vi "main.vi"() -> ()   [LabVIEW 2016]
uses:
  <userlib>/ROS for LabVIEW Software/ROS/Code/Console/Servers/ServerSubs/TopicDef.ctl
  <userlib>/ROS for LabVIEW Software/ROS/Code/SubVIs/_ROSDirection.ctl
  <userlib>/ROS for LabVIEW Software/ROS/MessageBuilding/std_msgs/subs/i8Scalar.vi
panel:
  in  "EM STOP":bool
  out "error out":errorcluster
  out "time":T1
  out "Error":cluster{"Error Code":i8, "Error Message":string}
  out "Ultrasonics":T2
  out "Lasers":T2
  in  "stop":bool
  out "Velocity":dbl
  out "Steering Angle":dbl(knob) scale=-20.0..20.0
  in  "settings":T3={"Enable"=0, "Run"=0, "GUI Connection"=1, "Max Speed"=3.0} {"Max Speed" min=0.5 max=10.0 step=0.25}
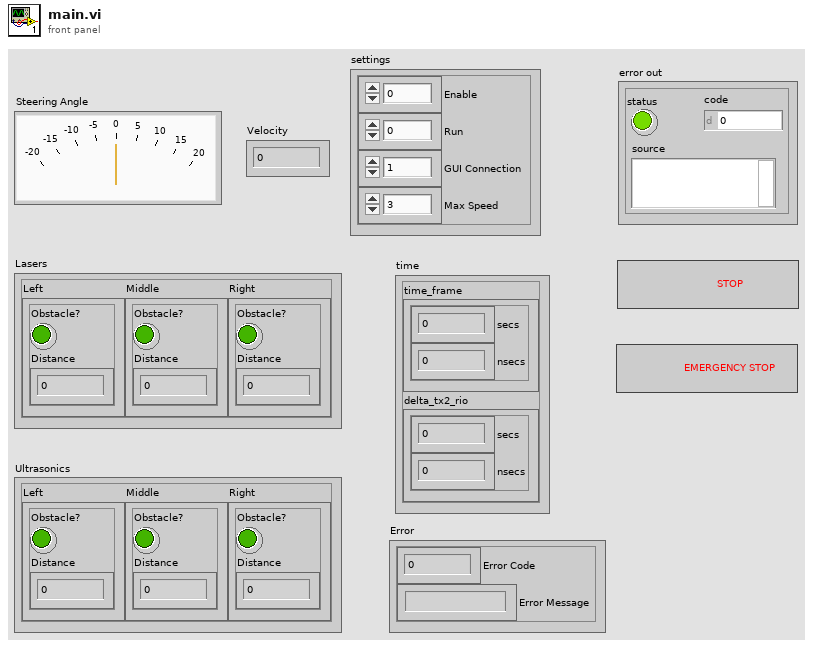
[diagram p1: front panel]
types:
  T1 = cluster{"time_frame":cluster{"secs":dbl, "nsecs":dbl}, "delta_tx2_rio":cluster{"secs":dbl, "nsecs":dbl}}
  T2 = cluster{"Left":cluster{"Obstacle?":bool, "Distance":dbl}, "Middle":cluster{"Obstacle?":bool, "Distance":dbl}, "Right":cluster{"Obstacle?":bool, "Distance":dbl}}
  T3 = cluster{"Enable":i8, "Run":i8, "GUI Connection":i8, "Max Speed":dbl}
  T4 = typedef "TopicDef.ctl" = cluster{"Topic":string, "Type":string, "Action":T5, "Update (ms)":u16, "queue size":u16}
  T5 = typedef "_ROSDirection.ctl" = enum16{"Node", "Publisher", "Subscriber", "ServiceClient", "ServiceProvider"}
  T6 = typedef "_ROSControl.ctl" = cluster{"topic port":u16, "Node":string, "topic":string, "type":string, "node port":u16, "error ":errorcluster, "Direction":T5, "Update (ms)":u16, "FIFO size":u16}
  T7 = cluster{"time_frame":cluster{"secs":i32, "nsecs":i32}, "delta_tx2_rio":cluster{"secs":i32, "nsecs":i32}}
  T8 = cluster{"speed_is":cluster{"steering_front_left":dbl, "steering_front_right":dbl, "steering_rear_left":dbl, "steering_rear_right":dbl}, "steering_is":cluster{"steering_front_left":dbl, "steering_front_right":dbl, "steering_rear_left":dbl, "steering_rear_right":dbl}, "distance_front":cluster{"left":dbl, "middle":dbl, "right":dbl}, "distance_back":cluster{"left":dbl, "middle":dbl, "right":dbl}, "error_id":i8, "error_message":string, "time_frame":cluster{"secs":i32, "nsecs":i32}, "delta_tx2_rio":cluster{"secs":i32, "nsecs":i32}}
  T9 = cluster{"steering_front_left":dbl, "steering_front_right":dbl, "steering_rear_left":dbl, "steering_rear_right":dbl}
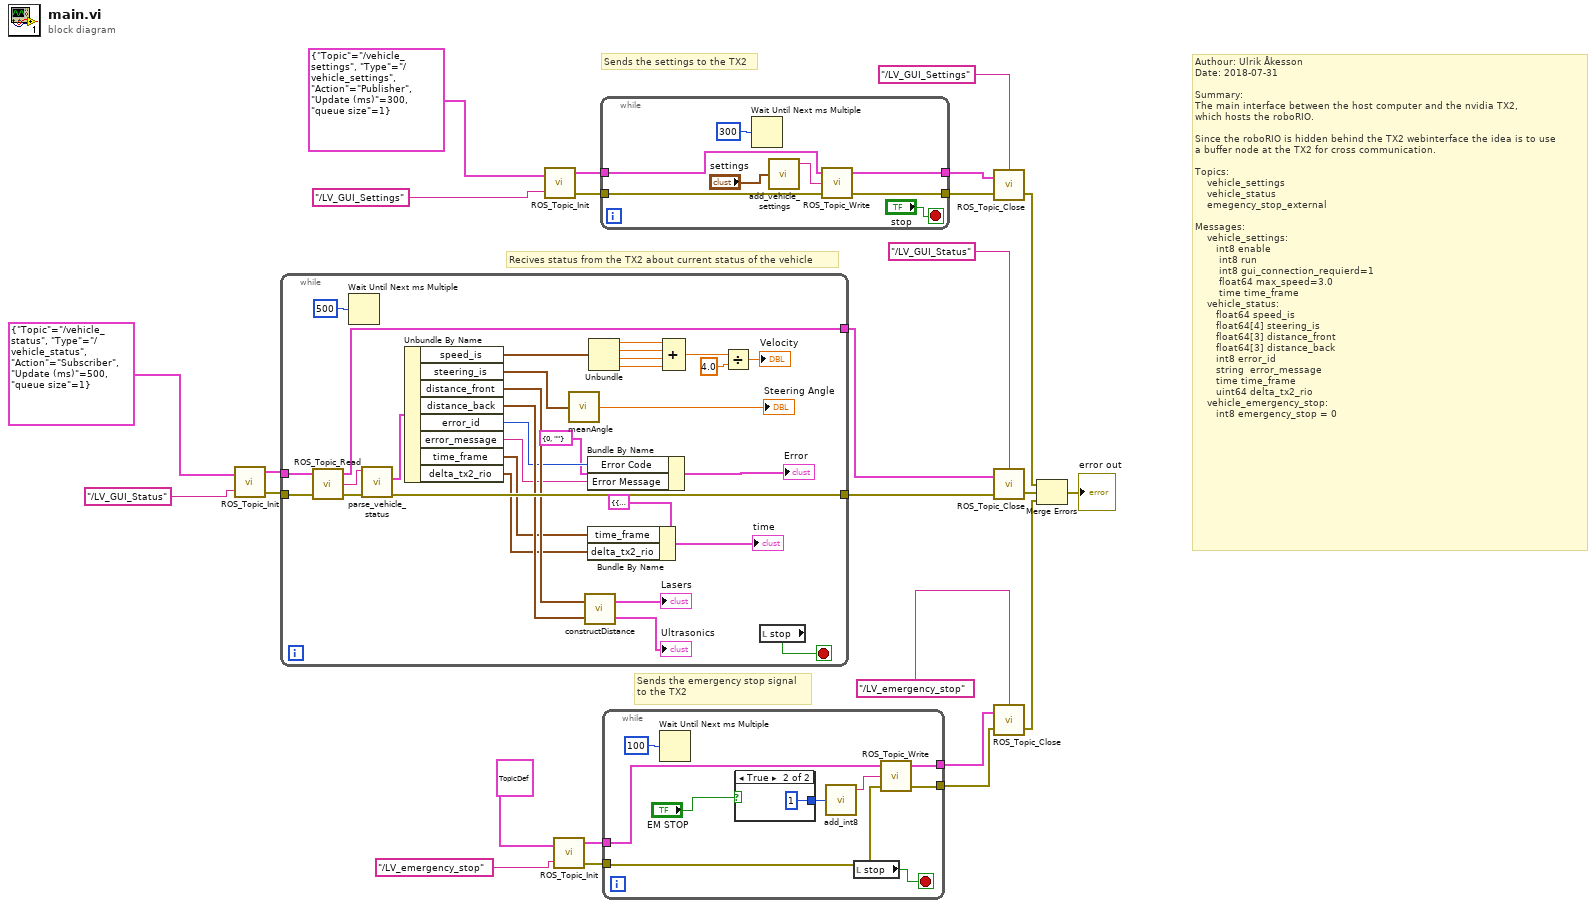
[diagram p0: block diagram]
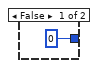
[diagram p2: hidden frame]
diagram:
  # "Sends the emergency stop signal\nto the TX2"
  # "Recives status from the TX2 about current status of the vehicle"
  # "Sends the settings to the TX2"
  # "Authour: Ulrik Åkesson\nDate: 2018-07-31\n\nSummary:\nThe main interface between the host computer and the nvidia TX2,\nwhich hosts the roboRIO.\n\nSince the roboRIO is hidden behind the TX2 webinterface the idea is to use\na buffer node at the TX2 for cross communication.\n\nTopics:\n    vehicle_settings\n    vehicle_status\n    emegency_stop_external\n\nMessages:\n    vehicle_settings:\n       int8 enable\n        int8 run\n        int8 gui_connection_requierd=1\n        float64 max_speed=3.0\n        time time_frame \n    vehicle_status:\n       float64 speed_is\n       float64[4] steering_is\n       float64[3] distance_front\n       float64[3] distance_back\n       int8 error_id\n       string  error_message\n       time time_frame\n       uint64 delta_tx2_rio\n    vehicle_emergency_stop:\n       int8 emergency_stop = 0"
  n1 = call <userlib>:"ROS_Topic_Init.vi"("Definitions"=T4 {"Topic"="/vehicle_status", "Type"="/vehicle_status", "Action"=enum."Subscriber", "Update (ms)"=500, "queue size"=1}, "node"="/LV_GUI_Status") -> ("ROS out"=w16:T6, "error out"=w15:errorcluster)  [unwired: 1 in]
  n2 = while {
    tunnel: w16 -> [w56]
    tunnel: w15 -> [w55]
    tunnel: [w50] -> w13
    tunnel: [w51] -> w12
    stop <- w49 stop-if-true
    n3 = call <userlib>:"ROS_Topic_Read.vi"("error in (no error)"=w55, "ROS in"=w56) -> ("error out"=w53:errorcluster, "Reply"=w54:string, "ROS out"=w50:T6)  [unwired: 1 in]
    n4 = Wait Until Next ms Multiple(millisecond multiple=u32 500) -> ()  [unwired: 1 out]
    n5 = call "parse_vehicle_status.vi"("error in"=w53, "msg in"=w54) -> ("error out"=w51:errorcluster, "vehicle_status"=w52:T8)  [unwired: 7 in, 1 out]
    n6 = Unbundle By Name(w52) -> ("speed_is"=w33:T9, "steering_is"=w47:T9, "distance_front"=w46:cluster{"left":dbl, "middle":dbl, "right":dbl}, "distance_back"=w45:cluster{"left":dbl, "middle":dbl, "right":dbl}, "error_id"=w42:i8, "error_message"=w41:string, "time_frame"=w37:cluster{"secs":i32, "nsecs":i32}, "delta_tx2_rio"=w36:cluster{"secs":i32, "nsecs":i32})
    n7 = call "meanAngle.vi"("steering_is"=w47) -> ("Numeric"=→"Steering Angle":dbl)
    n8 = call "constructDistance.vi"("distance_front"=w45, "distance_back"=w46) -> ("Ultrasonics"=→"Ultrasonics":T2, "Lasers"=→"Lasers":T2)
    n9 = Bundle By Name(cluster=cluster{"Error Code":i8, "Error Message":string} {"Error Code"=0, "Error Message"=""} ("Error 2"), "Error Code"=w42, "Error Message"=w41) -> (→"Error":cluster{"Error Code":i8, "Error Message":string})
    n10 = Bundle By Name(cluster=T7 {"time_frame"={"secs"=0, "nsecs"=0}, "delta_tx2_rio"={"secs"=0, "nsecs"=0}}, "time_frame"=w37, "delta_tx2_rio"=w36) -> (→"time":T7)
    n11 = Unbundle(w33) -> ("steering_front_left"=w32:dbl, "steering_front_right"=w31:dbl, "steering_rear_left"=w30:dbl, "steering_rear_right"=w29:dbl)
    n12 = Compound Arithmetic op=ADD(w32, w31, w30, w29) -> (w27:dbl)
    n13 = Divide(x=w27, y=4.0) -> (x/y=→"Velocity":dbl)
    n14 = local read "stop"() -> (w49:bool)
  }
  n15 = call <userlib>:"ROS_Topic_Init.vi"("Definitions"=T4 {"Topic"="/vehicle_settings", "Type"="/vehicle_settings", "Action"=enum."Publisher", "Update (ms)"=300, "queue size"=1}, "node"="/LV_GUI_Settings") -> ("ROS out"=w24:T6, "error out"=w23:errorcluster)  [unwired: 1 in]
  n16 = call <userlib>:"ROS_Topic_Init.vi"("Definitions"=T4 {"Topic"="/emergency_stop_external", "Type"="/vehicle_emergency_stop", "Action"=enum."Publisher", "Update (ms)"=100, "queue size"=1}, "node"="/LV_emergency_stop") -> ("ROS out"=w7:T6, "error out"=w6:errorcluster)  [unwired: 1 in]
  n17 = while {
    tunnel: w24 -> [w62]
    tunnel: w23 -> [w61]
    tunnel: [w59] -> w22
    tunnel: [w58] -> w21
    stop <- "stop" stop-if-true
    n18 = Wait Until Next ms Multiple(millisecond multiple=u32 300) -> ()  [unwired: 1 out]
    n19 = call "add_vehicle_settings.vi"("vehicle_settings"="settings") -> ("msg out"=w63:string)  [unwired: 4 in]
    n20 = call <userlib>:"ROS_Topic_Write.vi"("error in (no error)"=w61, "Msg in"=w63, "ROS in"=w62) -> ("error out"=w58:errorcluster, "ROS out"=w59:T6)  [unwired: 1 in]
  }
  n21 = while {
    tunnel: w7 -> [w71]
    tunnel: w6 -> [w70]
    tunnel: [w69] -> w4
    tunnel: [w68] -> w3
    stop <- w73 stop-if-true
    n22 = Wait Until Next ms Multiple(millisecond multiple=u32 100) -> ()  [unwired: 1 out]
    n23 = case shown="True" "EM STOP" {
      tunnel: [i8 0 i8 1] -> w66
      frame False {
      }
      frame True {
      }
    }
    n24 = call-poly <userlib>:"add_int8.vi"("Numeric"=w66) -> ("msg out"=w72:string)  [unwired: 4 in]
    n25 = local read "stop"() -> (w73:bool)
    n26 = call <userlib>:"ROS_Topic_Write.vi"("error in (no error)"=w70, "Msg in"=w72, "ROS in"=w71) -> ("error out"=w69:errorcluster, "ROS out"=w68:T6)  [unwired: 1 in]
  }
  n27 = call <userlib>:"ROS_Topic_Close.vi"("error in"=w21, "ROS in"=w22, "node"="/LV_GUI_Settings") -> ("error out"=w11:errorcluster)  [unwired: 1 in]
  n28 = call <userlib>:"ROS_Topic_Close.vi"("error in"=w12, "ROS in"=w13, "node"="/LV_GUI_Status") -> ("error out"=w10:errorcluster)  [unwired: 1 in]
  n29 = call <userlib>:"ROS_Topic_Close.vi"("error in"=w4, "ROS in"=w3, "node"="/LV_emergency_stop") -> ("error out"=w8:errorcluster)  [unwired: 1 in]
  n30 = Merge Errors(w11, w10, w8) -> (→"error out":errorcluster)
